vi "ParseJSON.vi"(8 "error in":errorcluster, 10 "offset (0)":i32, 11 "JSON string":string) -> (0 "error out":errorcluster, 1 "Value":T1, 2 "offset out":i32, 3 "JSON string copy":string, 5 "Remaining":bool)   [LabVIEW 2020]
uses:
  <vilib>/regexp/Match Regular Expression.xnode
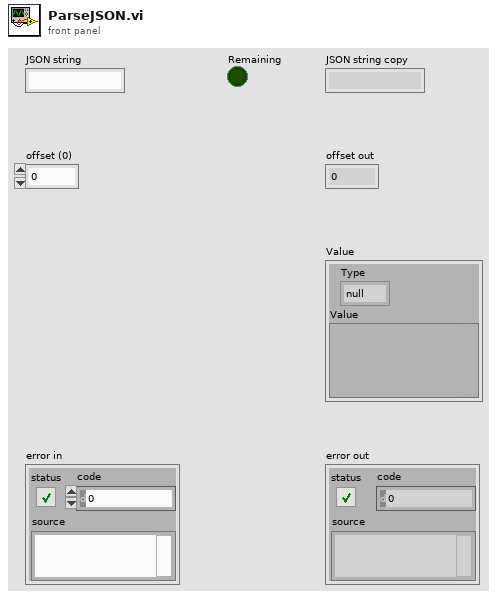
[diagram p1: front panel]
types:
  T1 = cluster{"Type":enum16{"null", "number", "boolean", "string", "array", "object", ""}, "Value":variant}
  T2 = cluster{"Key":string, "Value":cluster{"Type":enum16{"null", "number", "boolean", "string", "array", "object", ""}, "Value":variant}}
  T3 = enum16{"null", "number", "boolean", "string", "array", "object", ""}
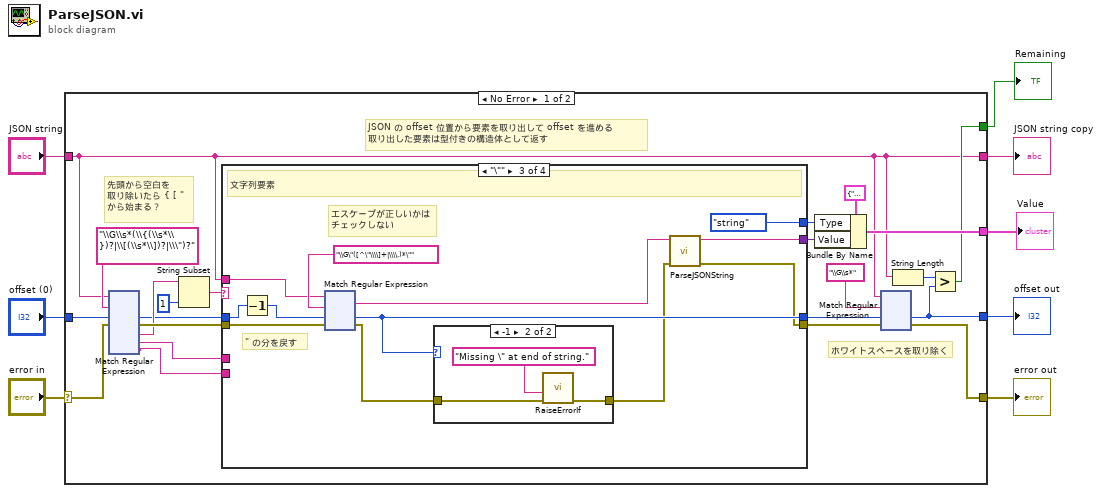
[diagram p0: block diagram]
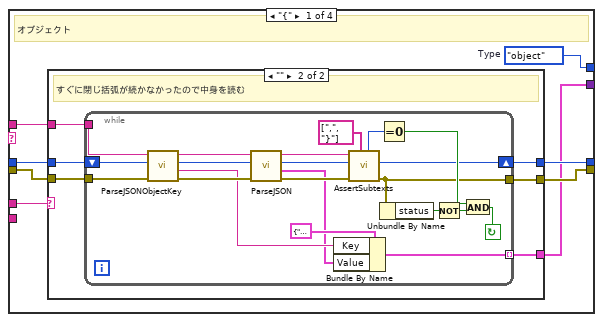
[diagram p2: hidden frame]
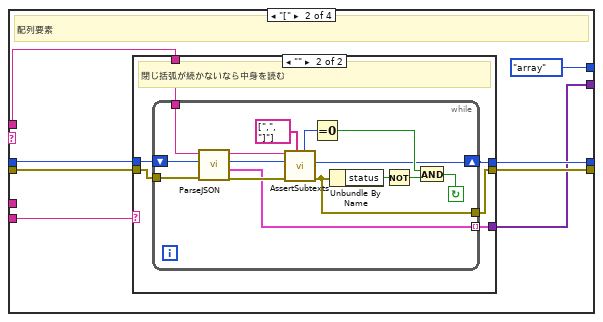
[diagram p4: hidden frame]
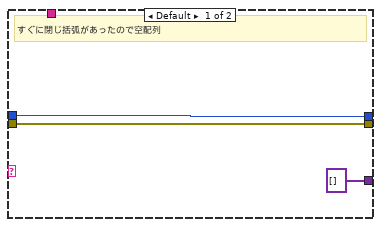
[diagram p5: hidden frame]
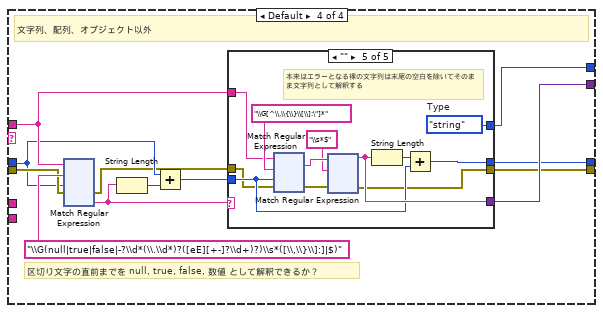
[diagram p7: hidden frame]
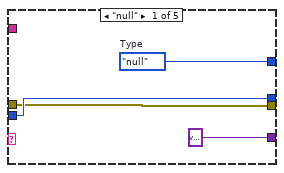
[diagram p8: hidden frame]
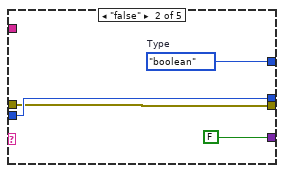
[diagram p9: hidden frame]
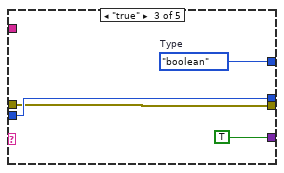
[diagram p10: hidden frame]
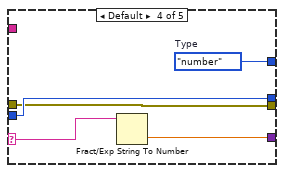
[diagram p11: hidden frame]
diagram:
  n1 = case shown="No Error" "error in" {
    selector: "error in" -> [w13 w867]
    tunnel: [w11 w865] -> w8
    tunnel: [w22 w867] -> w7
    tunnel: [w20 _] -> w6
    tunnel: "offset (0)" -> [w14 w865]
    tunnel: [w9 w866] -> w4
    tunnel: "JSON string" -> [w9 w866]
    tunnel: [w10 _] -> w1
    frame No Error {
      # "先頭から空白を\n取り除いたら { [ \" \nから始まる？"
      # "ホワイトスペースを取り除く"
      # "JSON の offset 位置から要素を取り出して offset を進める\n取り出した要素は型付きの構造体として返す"
      n2 = xnode "Match Regular Expression"("input string"=w9, "regular expression"="\\G\\s*(\\{(\\s*\\})?|\\[(\\s*\\])?|\\\")?", "offset (0)"=w14, "error in"=w13) -> ("offset past match"=w17:i32, "error out"=w26:errorcluster, "submatch 1"=w18:string, "submatch 2"=w16:string, "submatch 3"=w15:string)  [unwired: 2 in, 3 out]
      n3 = String Subset(string=w18, length (rest)=1 ("length (rest)")) -> (substring=w30:string)  [unwired: 1 in]
      n4 = case shown="\"\\\"\"" w30 {
        tunnel: [w274 w309 w346 w475] -> w25
        tunnel: [w273 w308 w343 w480] -> w28
        tunnel: w26 -> [w276 w311 w348 w481]
        tunnel: [w275 w310 w341 w471] -> w23
        tunnel: w17 -> [w270 w313 w340 w473]
        tunnel: w9 -> [w269 w312 w339 w477]
        tunnel: [w272 T3."array" ("Type") T3."string" w474] -> w21
        tunnel: w16 -> [w271 _ _ _]
        tunnel: w15 -> [_ w307 _ _]
        frame "{" {
          w272 = T3."object"  # Type
          # "オブジェクト"
          n5 = case shown="\"\"" w271 {
            tunnel: w276 -> [w278 w284]
            tunnel: w270 -> [w277 w283]
            tunnel: [w278 w282] -> w275
            tunnel: [_ w281] -> w273
            tunnel: [w277 w280] -> w274
            tunnel: w269 -> [_ w279]
            frame Default {
              # "すぐに閉じ括弧が続いたので空オブジェクト"
            }
            frame "" {
              # "すぐに閉じ括弧が続かなかったので中身を読む"
              n6 = while {
                tunnel: w284 -> [w305]
                tunnel: [w290] -> w281 mode=indexing
                shift-right: [w289] -> w280
                shift-left: w283 -> [w301]
                tunnel: [w288] -> w282
                tunnel: w279 -> [w285]
                stop <- w291 continue-if-true
                n7 = call "ParseJSONObjectKey.vi"("error in (no error)"=w305, "offset past match"=w301, "JSON string"=w285) -> ("error out"=w302:errorcluster, "key"=w287:string, "offset out"=w303:i32, "string copy"=w304:string)  [unwired: 5 in]
                n8 = call "ParseJSON.vi"("error in"=w302, "offset (0)"=w303, "JSON string"=w304) -> ("error out"=w300:errorcluster, "Value"=w286:T1, "offset out"=w299:i32, "JSON string copy"=w298:string)  [unwired: 4 in, 1 out]
                n9 = Bundle By Name(cluster=T2 {"Key"="", "Value"={"Type"=enum."null", "Value"=variant}}, "Key"=w287, "Value"=w286) -> (w290:T2)
                n10 = call "AssertSubtexts.vi"("Expected"=string[] [",", "}"], "error in"=w300, "offset"=w299, "string"=w298) -> ("error out"=w288:errorcluster, "offset out"=w289:i32, "Which found"=w295:i32)  [unwired: 4 in, 1 out]
                n11 = Equal To 0?(x=w295) -> (x = 0?=w292:bool)
                n12 = Unbundle By Name(w288) -> ("status"=w294:bool)
                n13 = Not(x=w294) -> (.not. x?=w293:bool)
                n14 = And(x=w292, y=w293) -> (x .and. y?=w291:bool)
              }
            }
          }
        }
        frame "[" {
          # "配列要素"
          n15 = case shown="\"\"" w307 {
            tunnel: w311 -> [w316 w322]
            tunnel: w312 -> [_ w321]
            tunnel: w313 -> [w314 w320]
            tunnel: [w316 w319] -> w310
            tunnel: [w314 w318] -> w309
            tunnel: [variant[] [] w317] -> w308
            frame Default {
              # "すぐに閉じ括弧があったので空配列"
            }
            frame "" {
              # "閉じ括弧が続かないなら中身を読む"
              n16 = while {
                tunnel: w322 -> [w337]
                tunnel: w321 -> [w336]
                shift-right: [w328] -> w318
                shift-left: w320 -> [w335]
                tunnel: [w327] -> w319
                tunnel: [w323] -> w317 mode=indexing
                stop <- w329 continue-if-true
                n17 = call "ParseJSON.vi"("error in"=w337, "offset (0)"=w335, "JSON string"=w336) -> ("error out"=w324:errorcluster, "Value"=w323:T1, "offset out"=w325:i32, "JSON string copy"=w326:string)  [unwired: 4 in, 1 out]
                n18 = call "AssertSubtexts.vi"("Expected"=string[] [",", "]"], "error in"=w324, "offset"=w325, "string"=w326) -> ("error out"=w327:errorcluster, "offset out"=w328:i32, "Which found"=w333:i32)  [unwired: 4 in, 1 out]
                n19 = Equal To 0?(x=w333) -> (x = 0?=w330:bool)
                n20 = Unbundle By Name(w327) -> ("status"=w332:bool)
                n21 = Not(x=w332) -> (.not. x?=w331:bool)
                n22 = And(x=w330, y=w331) -> (x .and. y?=w329:bool)
              }
            }
          }
        }
        frame "\"" {
          # "\" の分を戻す"
          # "エスケープが正しいかは\nチェックしない"
          # "文字列要素"
          n23 = Decrement(x=w340) -> (x-1=w338:i32)
          n24 = xnode "Match Regular Expression"("input string"=w339, "regular expression"="\\G\"([^\"\\\\]+|\\\\.)*\"", "offset (0)"=w338, "error in"=w348) -> ("whole match"=w344:string, "offset past match"=w346:i32, "error out"=w345:errorcluster)  [unwired: 2 in, 2 out]
          n25 = case shown="-1" w346 {
            tunnel: w345 -> [w350 w352]
            tunnel: [w350 w353] -> w342
            frame Default {
            }
            frame -1 {
              n26 = call "RaiseErrorIf.vi"("error in (no error)"=w352, "error message"="Missing \" at end of string." ("error source (\" \")")) -> ("error out"=w353:errorcluster)  [unwired: 9 in]
            }
          }
          n27 = call "ParseJSONString.vi"("error in (no error)"=w342, "JSON string"=w344) -> ("error out"=w341:errorcluster, "string"=w343:string)  [unwired: 8 in]
        }
        frame Default {
          # "区切り文字の直前までを null, true, false, 数値 として解釈できるか？"
          # "文字列、配列、オブジェクト以外"
          n28 = xnode "Match Regular Expression"("input string"=w477, "regular expression"="\\G(null|true|false|-?\\d*(\\.\\d*)?([eE][+-]?\\d+)?)\\s*([\\,\\}\\]:]|$)", "offset (0)"=w473, "error in"=w481) -> ("error out"=w472:errorcluster, "submatch 1"=w479:string)  [unwired: 2 in, 4 out]
          n29 = String Length(string=w479) -> (length=w478:i32)
          n30 = Add(x=w473, y=w478) -> (x+y=w476:i32)
          n31 = case shown="\"\"" w479 {
            selector: w479 -> [_ _ _ w497 _]
            tunnel: [variant ("Variant") FALSE TRUE w496 w507] -> w480
            tunnel: [w485 w490 w493 w499 w503] -> w474
            tunnel: w477 -> [_ _ _ _ w510]
            tunnel: w476 -> [w484 w488 w492 w498 w505]
            tunnel: [w484 w488 w492 w498 w504] -> w475
            tunnel: w472 -> [w483 w487 w491 w495 w502]
            tunnel: [w483 w487 w491 w495 w500] -> w471
            frame "null" {
              w485 = T3."null"  # Type
            }
            frame "false" {
              w490 = T3."boolean"  # Type
            }
            frame "true" {
              w493 = T3."boolean"  # Type
            }
            frame Default {
              w499 = T3."number"  # Type
              n32 = Fract/Exp String To Number(string=w497) -> (number=w496:dbl)  [unwired: 3 in, 1 out]
            }
            frame "" {
              w503 = T3."string"  # Type
              # "本来はエラーとなる裸の文字列は末尾の空白を除いてそのまま文字列として解釈する"
              n33 = xnode "Match Regular Expression"("input string"=w510, "regular expression"="\\G[^\\,\\{\\}\\[\\]:\"]*", "offset (0)"=w505, "error in"=w502) -> ("whole match"=w509:string, "error out"=w501:errorcluster)  [unwired: 2 in, 3 out]
              n34 = xnode "Match Regular Expression"("input string"=w509, "regular expression"="\\s*$", "error in"=w501) -> ("before match"=w507:string, "error out"=w500:errorcluster)  [unwired: 3 in, 3 out]
              n35 = String Length(string=w507) -> (length=w506:i32)
              n36 = Add(x=w506, y=w505) -> (x+y=w504:i32)
            }
          }
        }
      }
      n37 = Bundle By Name(cluster=T1 {"Type"=enum."null", "Value"=variant}, "Type"=w21, "Value"=w28) -> (w20:T1)
      n38 = xnode "Match Regular Expression"("input string"=w9, "regular expression"="\\G\\s*", "offset (0)"=w25, "error in"=w23) -> ("offset past match"=w11:i32, "error out"=w22:errorcluster)  [unwired: 2 in, 3 out]
      n39 = String Length(string=w9) -> (length=w12:i32)
      n40 = Greater?(x=w12, y=w11) -> (0:w10:bool)
    }
    frame Error {
    }
  }
  "offset out" <- w8
  "error out" <- w7
  "JSON string copy" <- w4
  "Value" <- w6
  "Remaining" <- w1
